vi "Mint e100 ActiveX example.vi"() -> ()   [LabVIEW 2015]
panel:
  in  "Run Motor 1":bool
  out "ADC 0 high":bool
  out "Waveform Chart":cluster{"Pos":sgl, "ADC":sgl, "ADC":sgl}(graph)
  in  "MintControls5560Lib.MintControllerCtrl":refnum<k7>(container)
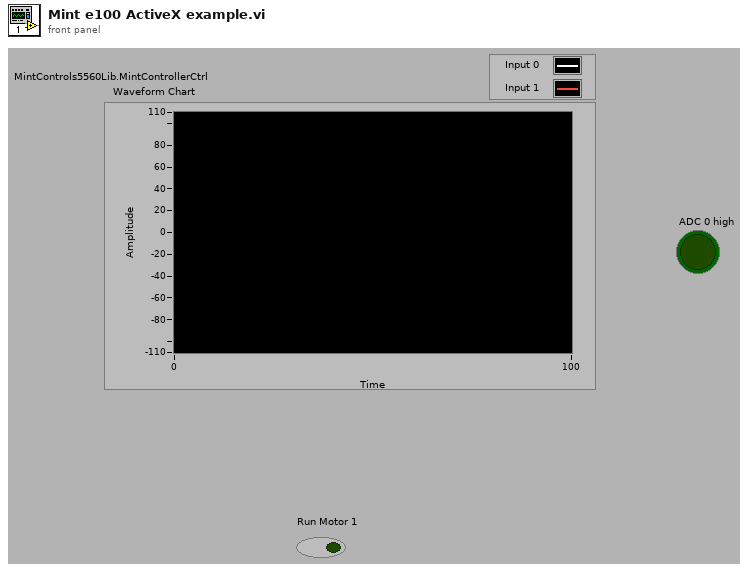
[diagram p1: front panel]
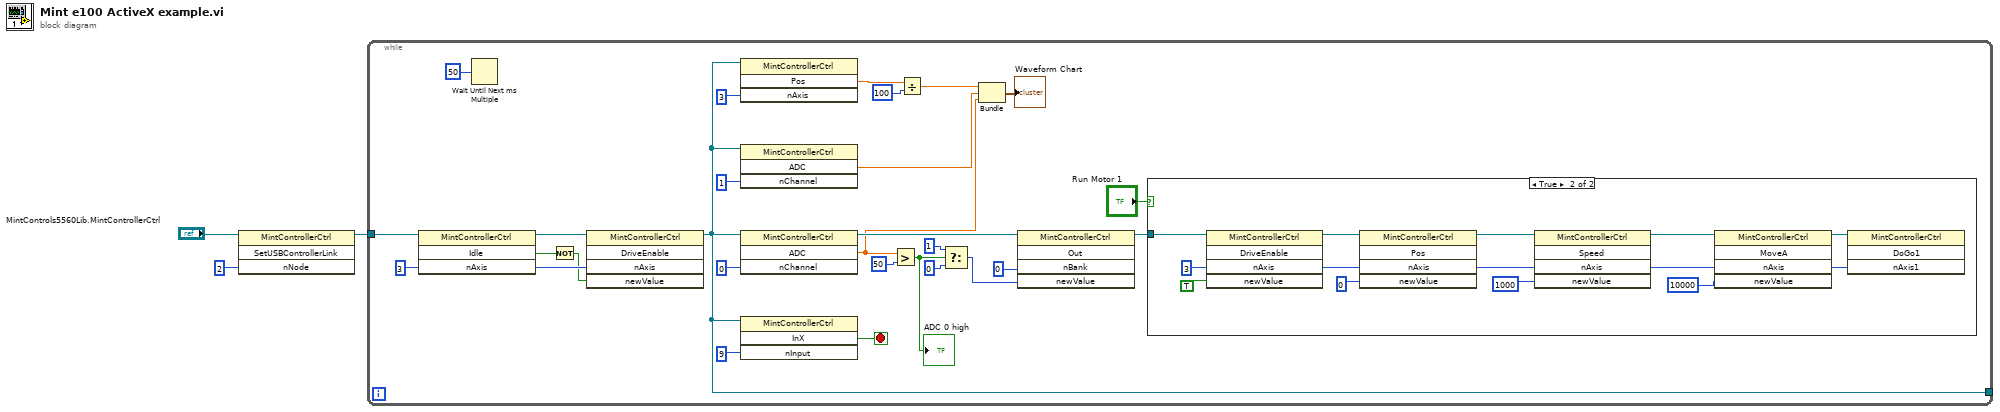
[diagram p0: block diagram]
diagram:
  n1 = invoke class="MintControllerCtrl" method="SetUSBControllerLink"(reference="MintControls5560Lib.MintControllerCtrl", "nNode"=2) -> (reference out=w1:refnum<k7>)  [unwired: 2 in, 3 out]
  n2 = while {
    tunnel: [w10] -> _
    tunnel: w1 -> [w9]
    stop <- w19 stop-if-true
    n3 = invoke class="MintControllerCtrl" method="Idle"(reference=w9, "nAxis"=3) -> (reference out=w8:refnum<k7>, "Idle"=w5:bool, "nAxis"=w7:i16)  [unwired: 2 in, 1 out]
    n4 = Wait Until Next ms Multiple(millisecond multiple=50) -> ()  [unwired: 1 out]
    n5 = Not(x=w5) -> (.not. x?=w4:bool)
    n6 = invoke class="MintControllerCtrl" method="DriveEnable"(reference=w8, "nAxis"=w7, "newValue"=w4) -> (reference out=w10:refnum<k7>)  [unwired: 2 in, 4 out]
    n7 = invoke class="MintControllerCtrl" method="Pos"(reference=w10, "nAxis"=3) -> ("Pos"=w17:sgl)  [unwired: 2 in, 3 out]
    n8 = invoke class="MintControllerCtrl" method="ADC"(reference=w10, "nChannel"=1) -> ("ADC"=w12:sgl)  [unwired: 2 in, 3 out]
    n9 = invoke class="MintControllerCtrl" method="ADC"(reference=w10, "nChannel"=0) -> (reference out=w15:refnum<k7>, "ADC"=w14:sgl)  [unwired: 2 in, 2 out]
    n10 = invoke class="MintControllerCtrl" method="InX"(reference=w10, "nInput"=9) -> ("InX"=w19:bool)  [unwired: 2 in, 3 out]
    n11 = Greater?(x=w14, y=50) -> (0:w23:bool)
    "ADC 0 high" <- w23
    n12 = Divide(x=w17, y=100) -> (x/y=w13:sgl)
    n13 = Select(t=1, s=w23, f=0) -> (s? t:f=w27:i32)
    n14 = Bundle(w13, "ADC"=w12, "ADC"=w14) -> (→"Waveform Chart":cluster{sgl, "ADC":sgl, "ADC":sgl})  [unwired: 1 in]
    n15 = invoke class="MintControllerCtrl" method="Out"(reference=w15, "nBank"=0, "newValue"=w27) -> (reference out=w20:refnum<k7>)  [unwired: 2 in, 4 out]
    n16 = case shown="True" "Run Motor 1" {
      tunnel: w20 -> [_ w42]
      frame False {
      }
      frame True {
        n17 = invoke class="MintControllerCtrl" method="DriveEnable"(reference=w42, "nAxis"=3, "newValue"=TRUE) -> (reference out=w34:refnum<k7>, "nAxis"=w33:i16)  [unwired: 2 in, 3 out]
        n18 = invoke class="MintControllerCtrl" method="Pos"(reference=w34, "nAxis"=w33, "newValue"=0) -> (reference out=w35:refnum<k7>, "nAxis"=w32:i16)  [unwired: 2 in, 3 out]
        n19 = invoke class="MintControllerCtrl" method="Speed"(reference=w35, "nAxis"=w32, "newValue"=1000) -> (reference out=w37:refnum<k7>, "nAxis"=w39:i16)  [unwired: 2 in, 3 out]
        n20 = invoke class="MintControllerCtrl" method="MoveA"(reference=w37, "nAxis"=w39, "newValue"=10000) -> (reference out=w44:refnum<k7>, "nAxis"=w40:i16)  [unwired: 2 in, 3 out]
        n21 = invoke class="MintControllerCtrl" method="DoGo1"(reference=w44, "nAxis1"=w40) -> ()  [unwired: 2 in, 4 out]
      }
    }
  }
